vi "getHPBroadcastCounter.vi"(11 "ILCCommunications in":refnum<class "ILCCommunications.lvclass">) -> (2 "HPBroadcastCounter":u8, 3 "ILCCommunications out":refnum<class "ILCCommunications.lvclass">)   [LabVIEW 2016]
uses:
  ILCCommunications.lvclass
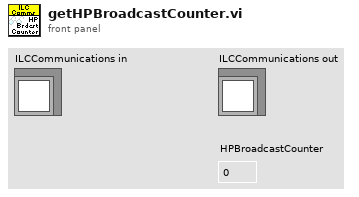
[diagram p1: front panel]
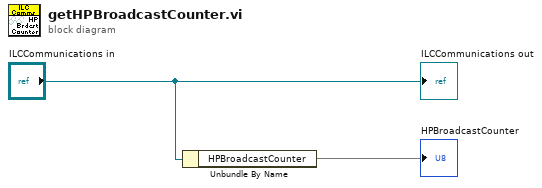
[diagram p0: block diagram]
diagram:
  n1 = Unbundle By Name("ILCCommunications in") -> ("HPBroadcastCounter"=→"HPBroadcastCounter")
  "ILCCommunications out" <- "ILCCommunications in"
